vi "FindMyBlueSerializableMethodPaths.vi"(8 "error in (no error)":errorcluster, 11 "LVClass refnum":refnum<vi>) -> (0 "error out":errorcluster, 1 "BlueSerialization Folder":path, 2 "BlueSerializable Paths":T1, 3 "LVClass refnum (dup)":refnum<vi>)   [LabVIEW 2019, in "BlueSerializationScripts.lvlib"]
uses:
  BlueSerializationScripts.lvlib
  BlueSerializableTemplatePaths.ctl
  BlueUtilityScripts/GetDescendantOptions.ctl
  2b3ae2fc-1e8e-41ba-8a56-12cdd7eb5315.vi
  2b3ae2fc-1e8e-41ba-8a56-12cdd7eb5315.vi/075dad69-f3ec-4759-863a-8144f738e76a.vi
  BlueSerialProviderGlobal.vi
  <userlib>/_OpenG.lib/file/file.llb/File Exists - Scalar__ogtk.vi
  <vilib>/Utility/error.llb/Error Cluster From Error Code.vi
  <vilib>/ErrorRing/Error Ring.xnode
  BlueUtilityScripts/BlueUtilityScripts.lvlib
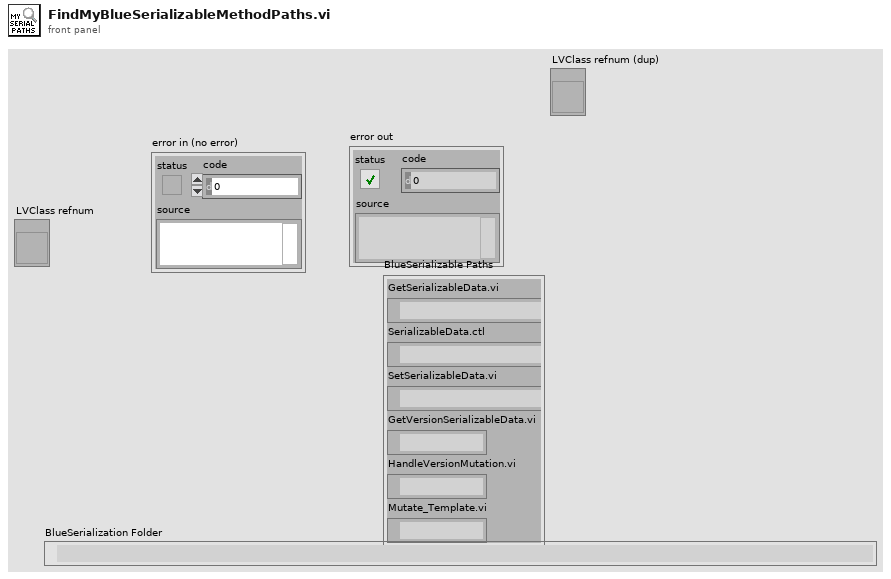
[diagram p1: front panel]
types:
  T1 = typedef "BlueSerializationScripts.lvlib/BlueSerializableTemplatePaths.ctl" = cluster{"GetSerializableData.vi":path, "SerializableData.ctl":path, "SetSerializableData.vi":path, "GetVersionSerializableData.vi":path, "HandleVersionMutation.vi":path, "Mutate_Template.vi":path}
  T2 = typedef "BlueUtilityScripts.lvlib/GetDescendantOptions.ctl" = cluster{"Type":string, "ExcludeDependencies":bool, "ExcludeBuilds":bool, "ExcludeTargets":bool}
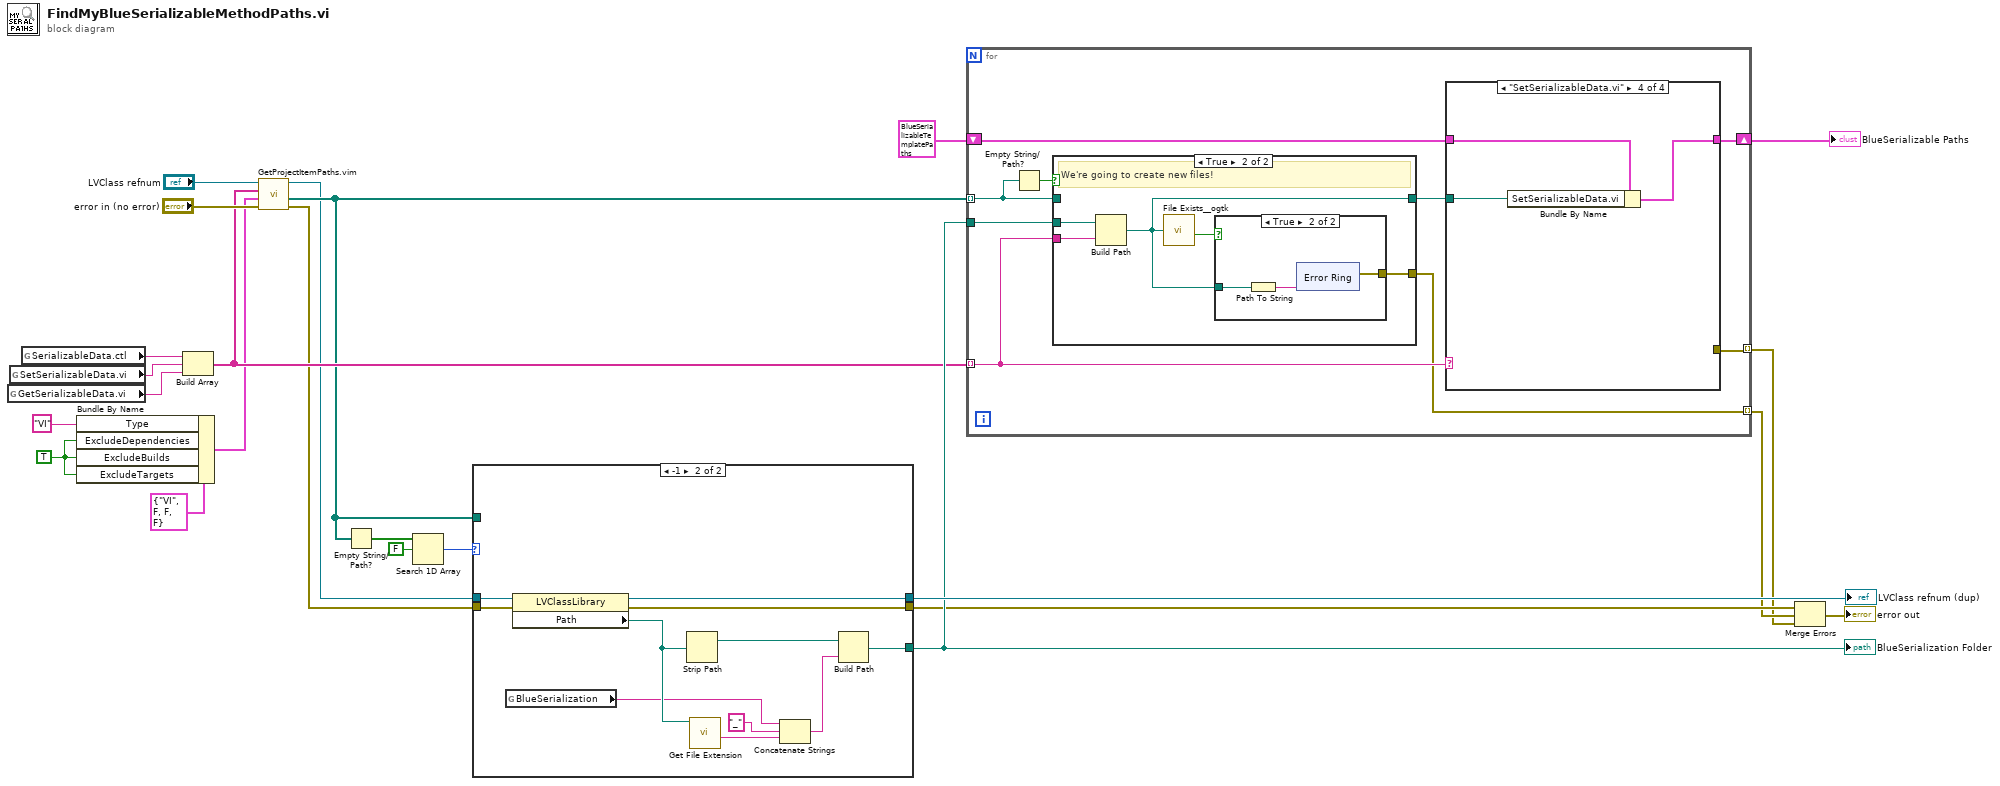
[diagram p0: block diagram]
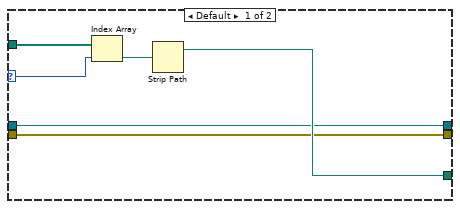
[diagram p2: hidden frame]
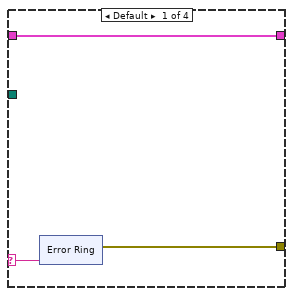
[diagram p5: hidden frame]
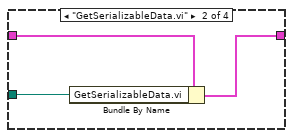
[diagram p6: hidden frame]
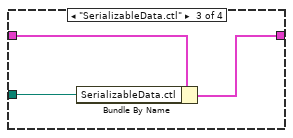
[diagram p7: hidden frame]
diagram:
  w8 = TRUE ("ExcludeBuilds")
  n1 = global read "BlueSerialProviderGlobal.vi" "GetSerializableData.vi"() -> (w3:string)
  n2 = global read "BlueSerialProviderGlobal.vi" "SetSerializableData.vi"() -> (w13:string)
  n3 = global read "BlueSerialProviderGlobal.vi" "SerializableData.ctl"() -> (w4:string)
  n4 = Bundle By Name(cluster=T2 {"Type"="VI", "ExcludeDependencies"=FALSE, "ExcludeBuilds"=FALSE, "ExcludeTargets"=FALSE} ("Search Options"), "Type"="VI", "ExcludeDependencies"=w8, "ExcludeBuilds"=w8, "ExcludeTargets"=w8) -> (w7:T2)
  n5 = Build Array(w4, w13, w3) -> (w12:string[])
  n6 = call "GetProjectItemPaths.vim"("error in (no error)"="error in (no error)", "Search Options"=w7, "Item Name"=w12, "ProjectItem"="LVClass refnum") -> ("error out"=w5:errorcluster, "Paths"=w6:path[], "ProjectItem"=w1:refnum<vi>)  [unwired: 4 in, 1 out]
  n7 = Empty String/Path?(string/path=w6) -> (empty?=w23:bool[])
  n8 = Search 1D Array(1D array=w23, element=FALSE) -> (index of element=w21:i32)  [unwired: 1 in]
  n9 = case shown="-1" w21 {
    selector: w21 -> [w29 _]
    tunnel: w6 -> [w30 _]
    tunnel: [w27 w38] -> w17
    tunnel: w1 -> [w26 w41]
    tunnel: [w25 w37] -> w16
    tunnel: [w26 w36] -> w18
    tunnel: w5 -> [w25 w35]
    frame Default {
      n10 = Index Array(array=w30, index=w29) -> (element=w28:path)
      n11 = Strip Path(path=w28) -> (stripped path=w27:path)  [unwired: 1 out]
    }
    frame -1 {
      n12 = global read "BlueSerialProviderGlobal.vi" "BlueSerialization"() -> (w34:string)
      n13 = property class="LVClassLibrary"(reference=w41, error in=w35) -> (reference out=w36:refnum<vi>, error out=w37:errorcluster, "Path"=w39:path)
      n14 = Strip Path(path=w39) -> (stripped path=w40:path)  [unwired: 1 out]
      n15 = call <vilib>:"Get File Extension.vi"("file"=w39) -> ("filename without extension"=w32:string)  [unwired: 6 in, 4 out]
      n16 = Concatenate Strings(w34, "_" ("string"), w32) -> (w31:string)
      n17 = Build Path(base path=w40, name or relative path=w31) -> (appended path=w38:path)
    }
  }
  "BlueSerialization Folder" <- w17
  "LVClass refnum (dup)" <- w18
  n18 = for {
    shift-right: [w49] -> w19
    shift-left: T1 {"GetSerializableData.vi"=path "", "SerializableData.ctl"=path "", "SetSerializableData.vi"=path "", "GetVersionSerializableData.vi"=path "", "HandleVersionMutation.vi"=path "", "Mutate_Template.vi"=path ""} ("BlueSerializableTemplate Paths") -> [w50]
    tunnel: w6 -> [w47] mode=indexing
    tunnel: w12 -> [w45] mode=indexing
    tunnel: w17 -> [w46]
    tunnel: [w43] -> w15 mode=indexing
    tunnel: [w42] -> w11 mode=indexing
    n19 = Empty String/Path?(string/path=w47) -> (empty?=w48:bool)
    n20 = case shown="True" w48 {
      tunnel: w47 -> [w51 _]
      tunnel: w46 -> [_ w56]
      tunnel: w45 -> [_ w55]
      tunnel: [w51 w53] -> w44
      tunnel: [_ w52] -> w43
      frame False {
        # "File already exists and is in our class library"
      }
      frame True {
        # "We're going to create new files!"
        n21 = Build Path(base path=w56, name or relative path=w55) -> (appended path=w53:path)
        n22 = call-poly <userlib>:"File Exists__ogtk.vi"("file path"=w53) -> ("exists"=w54:bool)  [unwired: 6 in, 1 out]
        n23 = case shown="True" w54 {
          tunnel: w53 -> [_ w58]
          tunnel: [_ w57] -> w52
          frame False {
          }
          frame True {
            n24 = Path To String(path=w58) -> (string=w59:string)
            n25 = xnode "Error Ring"("parameter 0"=w59) -> ("error out"=w57:errorcluster)
          }
        }
      }
    }
    n26 = case shown="\"SetSerializableData.vi\"" w45 {
      selector: w45 -> [w68 _ _ _]
      tunnel: w50 -> [w69 w79 w82 w85]
      tunnel: w44 -> [_ w78 w81 w84]
      tunnel: [w69 w77 w80 w83] -> w49
      tunnel: [w67 _ _ _] -> w42
      frame Default {
        n27 = xnode "Error Ring"("parameter 0"=w68) -> ("error out"=w67:errorcluster)
      }
      frame "GetSerializableData.vi" {
        n28 = Bundle By Name(cluster=w79, "GetSerializableData.vi"=w78) -> (w77:T1)
      }
      frame "SerializableData.ctl" {
        n29 = Bundle By Name(cluster=w82, "SerializableData.ctl"=w81) -> (w80:T1)
      }
      frame "SetSerializableData.vi" {
        n30 = Bundle By Name(cluster=w85, "SetSerializableData.vi"=w84) -> (w83:T1)
      }
    }
  }
  "BlueSerializable Paths" <- w19
  n31 = Merge Errors(w16, w15, w11) -> (→"error out":errorcluster)
